vi "Reset Timer.vi"(8 "error in (no error)":errorcluster, 11 "UI_ProgressBar in":refnum<class "UI_ProgressDlg.lvclass">) -> (0 "error out":errorcluster, 3 "UI_ProgressBar out":refnum<class "UI_ProgressDlg.lvclass">)   [LabVIEW 2014, in "UI_ProgressDlg.lvlib" / "UI_ProgressDlg.lvclass"]
uses:
  UI_ProgressDlg.lvclass
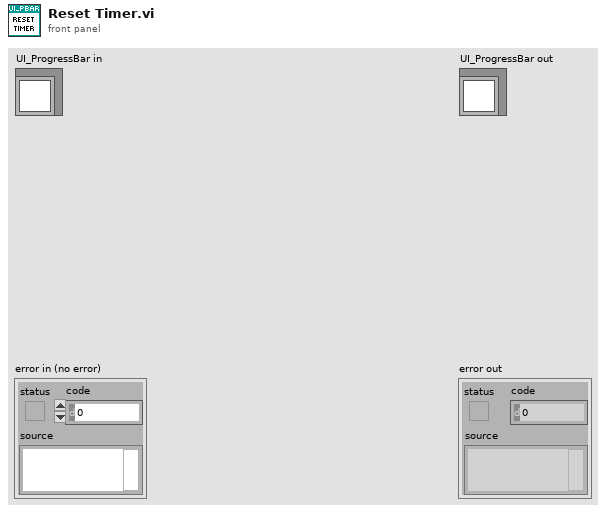
[diagram p1: front panel]
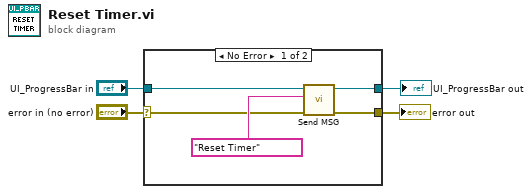
[diagram p0: block diagram]
diagram:
  n1 = case shown="No Error" "error in (no error)" {
    selector: "error in (no error)" -> [w5 w11]
    tunnel: [w8 w11] -> w3
    tunnel: [w9 w10] -> w1
    tunnel: "UI_ProgressBar in" -> [w7 w10]
    frame No Error {
      n2 = call "Send MSG.vi"("error in (no error)"=w5, "msg"="Reset Timer" ("Inforamtion"), "UI_ProgressBar in"=w7) -> ("error out"=w8:errorcluster, "UI_ProgressBar out"=w9:refnum<class "UI_ProgressDlg.lvclass">)  [unwired: 7 in]
    }
    frame Error {
    }
  }
  "error out" <- w3
  "UI_ProgressBar out" <- w1
